vi "main_nova.vi"() -> ()   [LabVIEW 2019]
panel:
  out "error out 3":errorcluster
  in  "MoveL":bool
  out "DigitalOutput":u8[](array[numeric])
  out "DigitalInput":u8[](array[numeric])
  out "Current SpeedFactor":dbl
  out "error out 2":errorcluster
  in  "Digital Outputs Index:":i32=1 min=1 max=16 step=1
  out "Error Log":string
  in  "GetErrorID":bool
  out "x value":string
  out "y value":string
  out "z value":string
  out "rx value":string
  out "ry value":string
  out "rz value":string
  out "j6 value":string
  out "j5 value":string
  out "j4 value":string
  out "j3 value":string
  out "j2 value":string
  out "j1 value":string
  in  "rz-":bool
  in  "ry-":bool
  in  "rx-":bool
  in  "z-":bool
  in  "y-":bool
  in  "x-":bool
  in  "rz+":bool
  in  "ry+":bool
  in  "rx+":bool
  in  "z+":bool
  in  "y+":bool
  in  "x+":bool
  in  "j6":dbl
  in  "j5":dbl
  in  "j4":dbl
  in  "j3":dbl
  in  "j2":dbl
  in  "j1":dbl
  in  "Set IO confrim":bool
  in  "Status":string(combo)="1"
  in  "Feedback Port":string="30004"
  in  "Dashboard Port":string="29999"
  in  "IP Address":string="192.168.5.1"
  in  "stop get state":bool
  out "state error out 2":errorcluster
  out "Robot mode":T1(ring)
  out "speed set string":string
  in  "j6-":bool
  in  "j5-":bool
  in  "j4-":bool
  in  "j3-":bool
  in  "j2-":bool
  in  "j1-":bool
  in  "j6+":bool
  in  "j5+":bool
  in  "j4+":bool
  in  "j3+":bool
  in  "j2+":bool
  in  "j1+":bool
  in  "stop connect":bool
  in  "Start trace":bool
  in  "tracePath":string
  in  "Stop move":bool
  in  "MoveJ":bool
  in  "rz":dbl
  in  "ry":dbl
  in  "rx":dbl
  in  "z":dbl
  in  "y":dbl
  in  "x":dbl
  in  "Speed confrim":bool
  in  "Speed Ratio":dbl=50.0
  in  "Emergency Stop":bool
  in  "Power up":bool
  out "Log":string
  in  "ClearError":bool
  in  "Enable Robot":bool
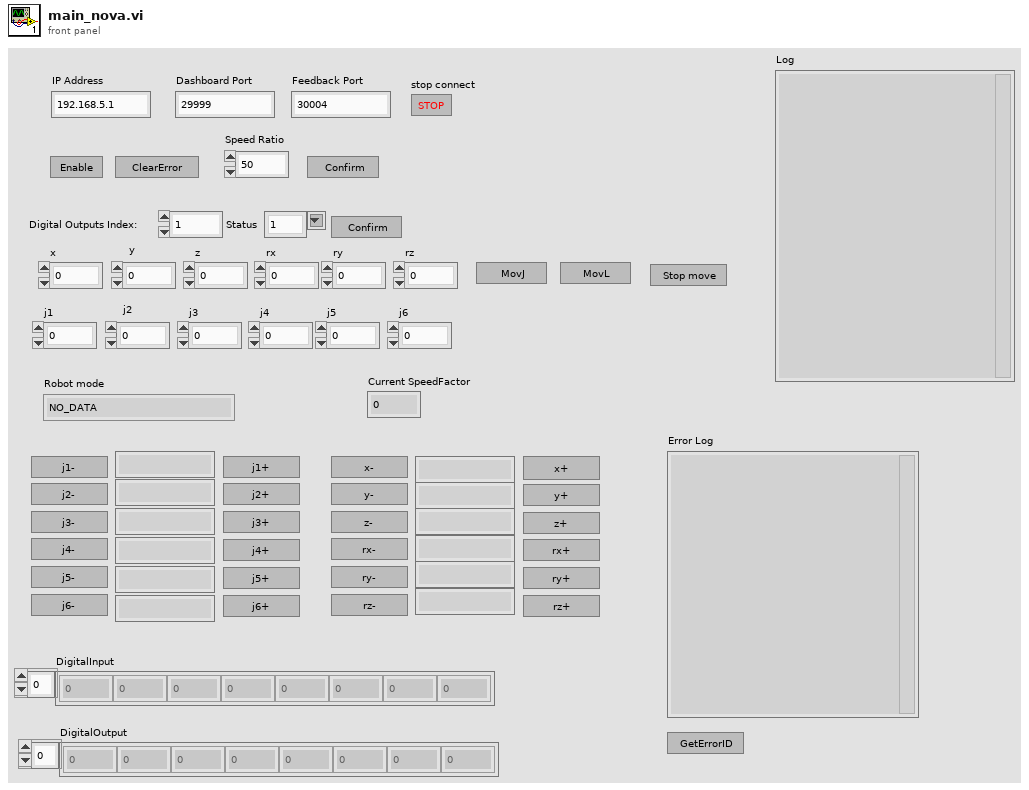
[diagram p1: front panel]
types:
  T1 = enum16{"NO_DATA", "ROBOT_MODE_INIT", "ROBOT_MODE_BRAKE_OPEN", "HOLD_BITS", "ROBOT_MODE_DISABLED", "ROBOT_MODE_ENABLE", "ROBOT_MODE_BACKDRIVE", "ROBOT_MODE_RUNNING", "ROBOT_MODE_RECORDING", "ROBOT_MODE_ERROR", "ROBOT_MODE_PAUSE", "ROBOT_MODE_JOG"}
  T2 = enum16{"Standard", "Buffered", "CRLF", "Immediate"}
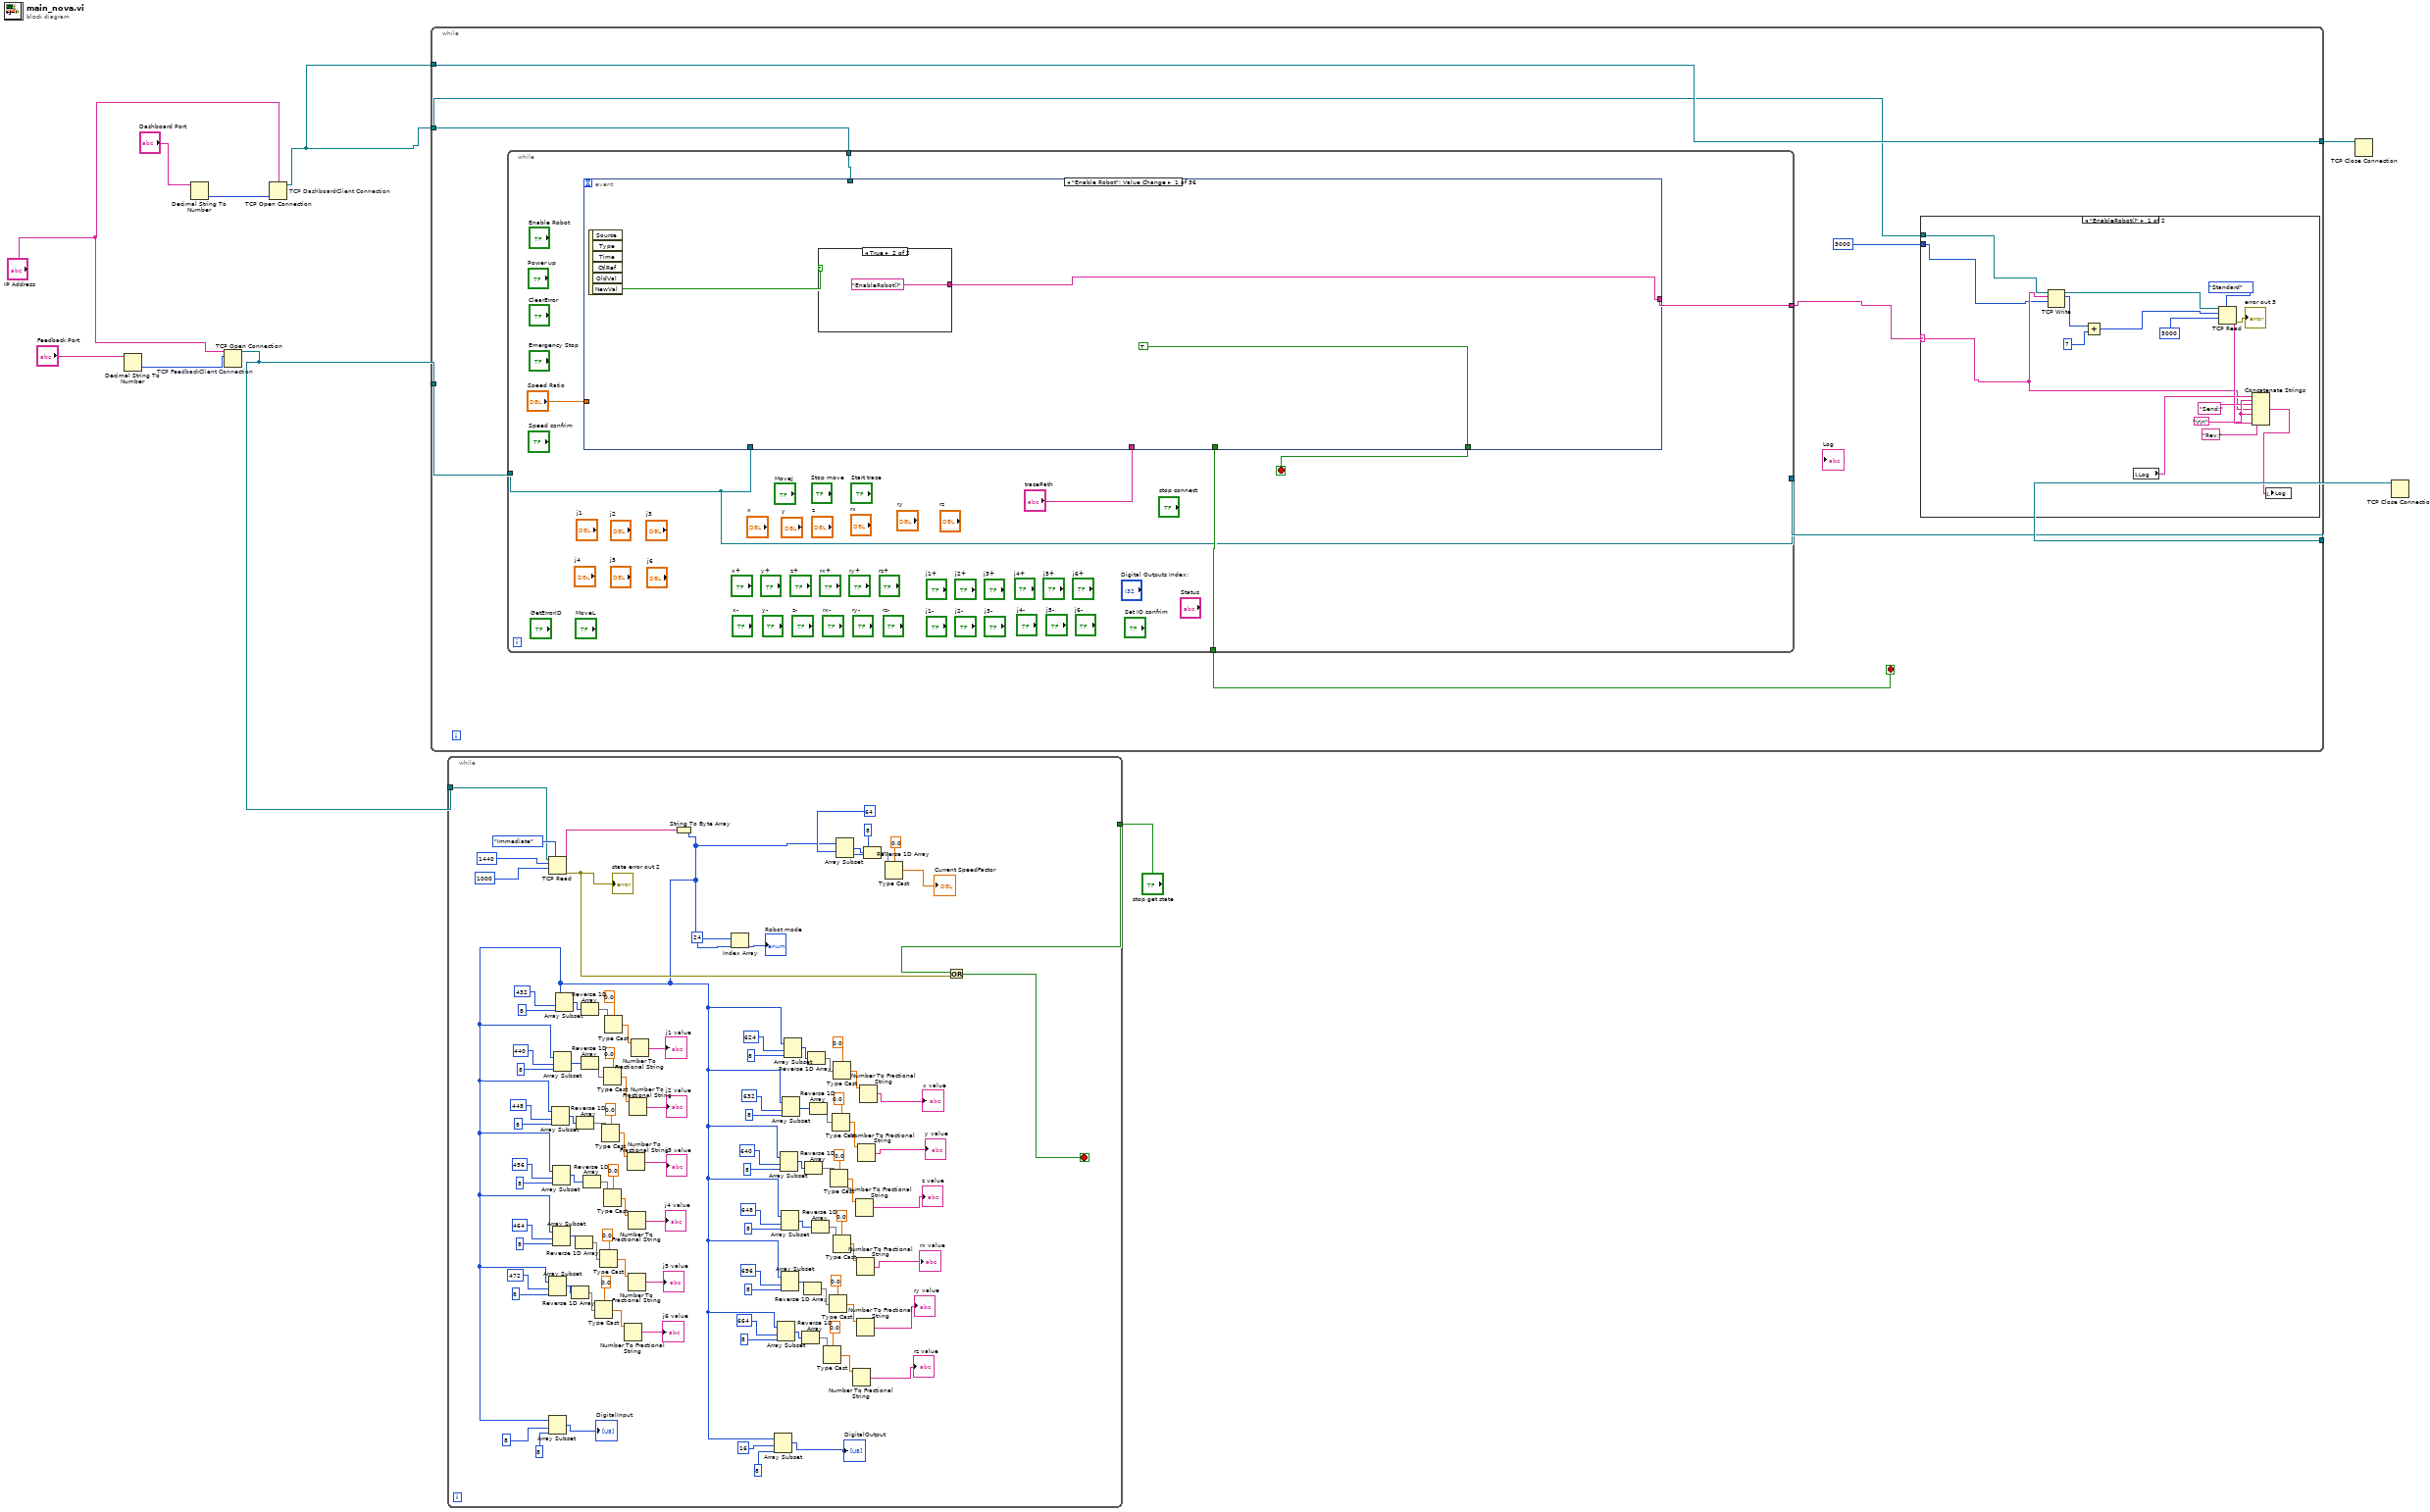
[diagram p0: block diagram]
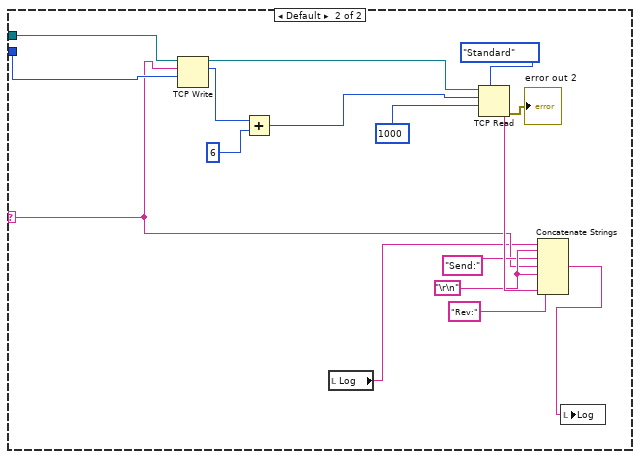
[diagram p2: hidden frame]
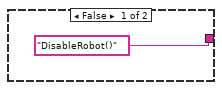
[diagram p3: hidden frame]
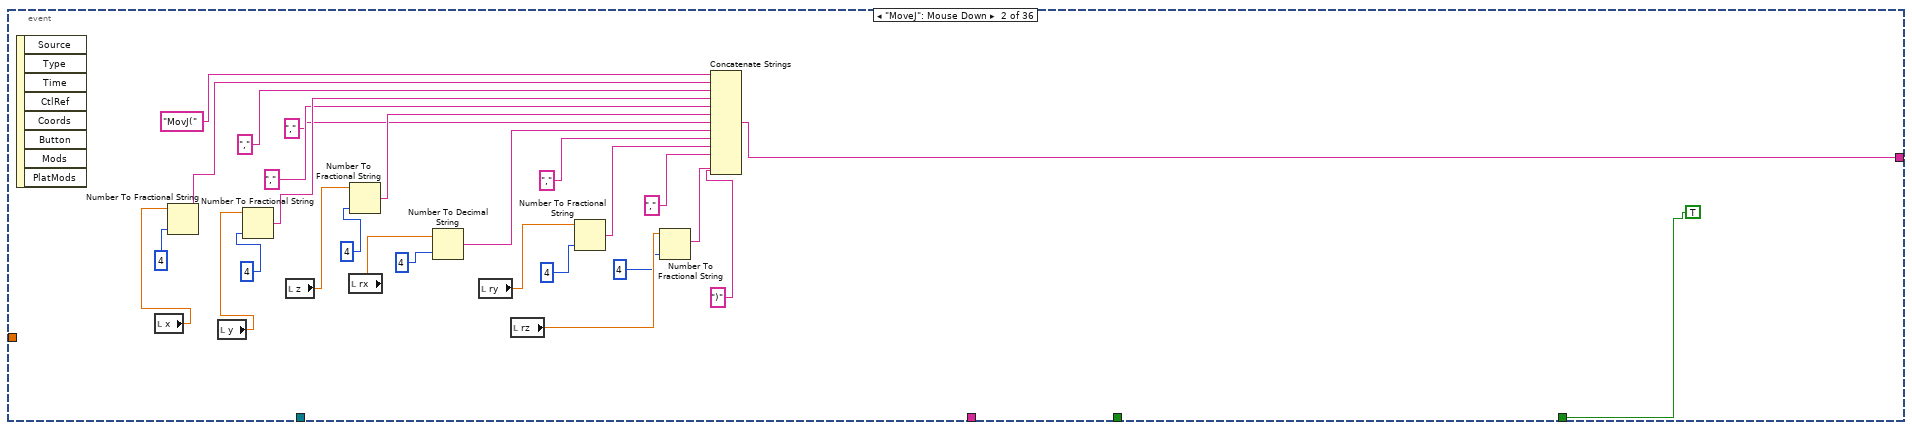
[diagram p4: hidden frame]
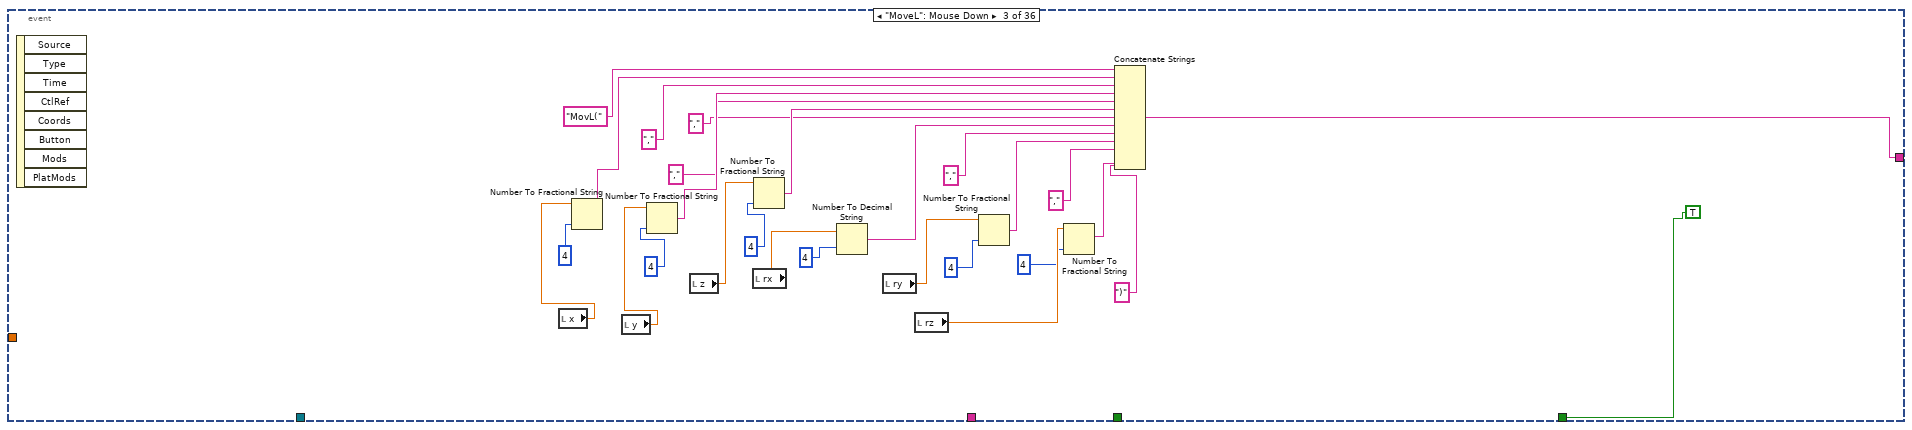
[diagram p5: hidden frame]
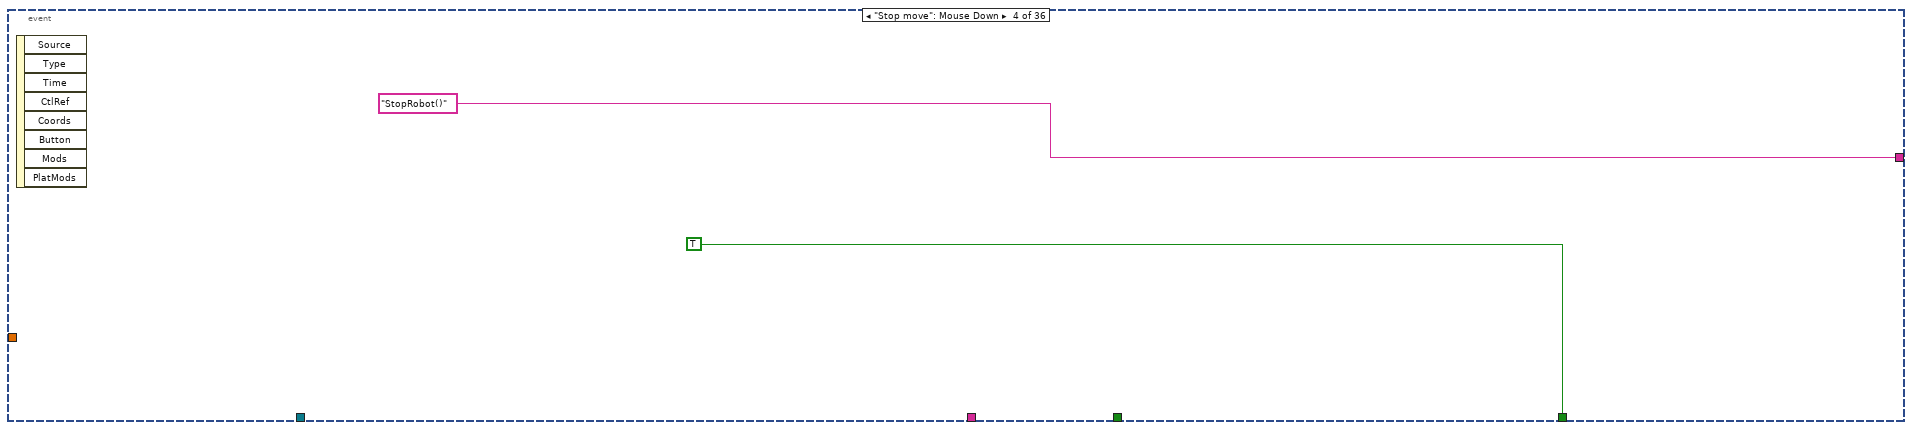
[diagram p6: hidden frame]
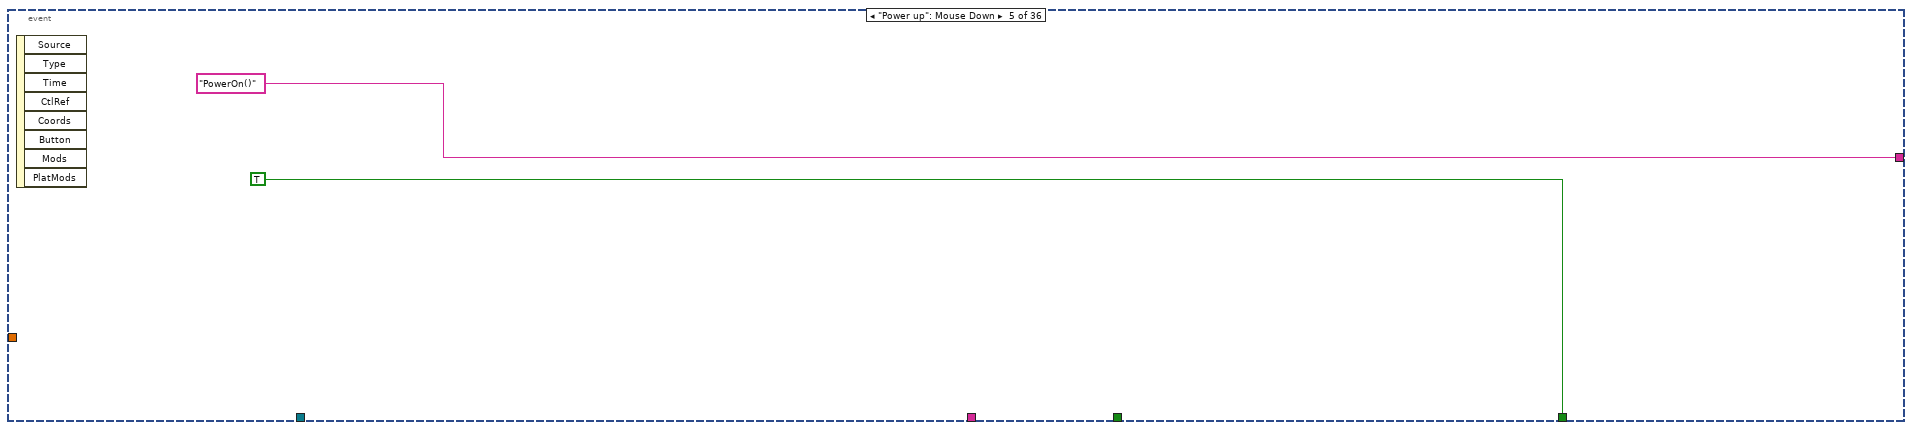
[diagram p7: hidden frame]
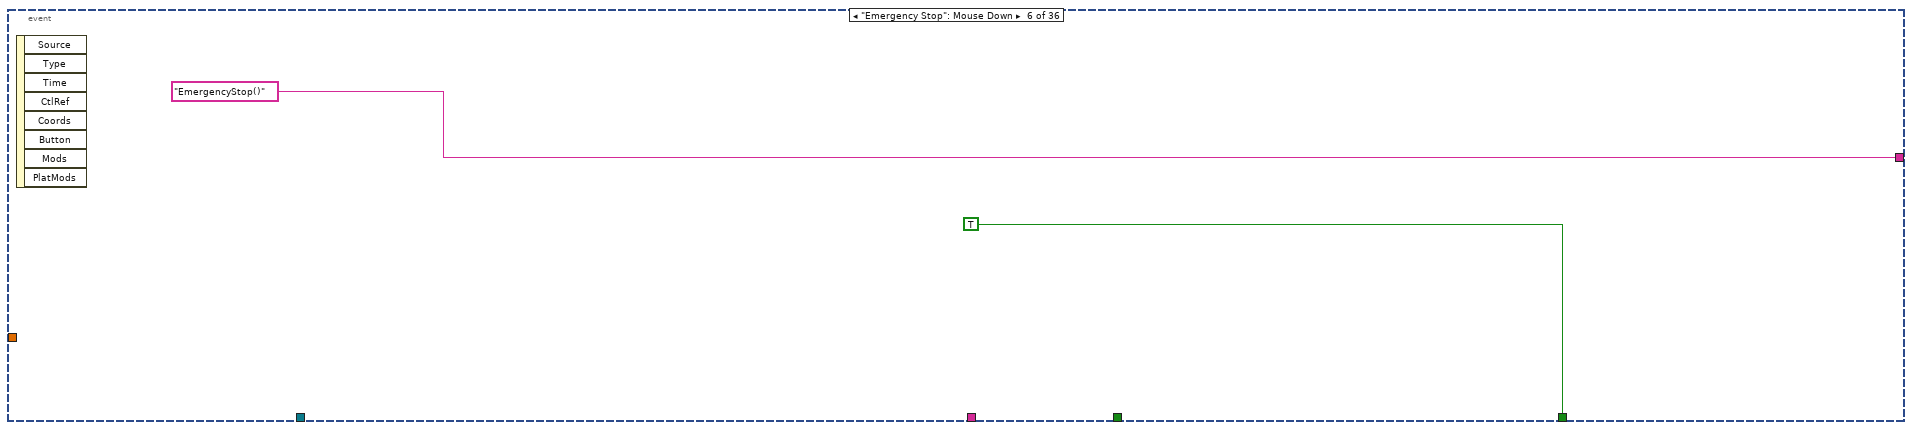
[diagram p8: hidden frame]
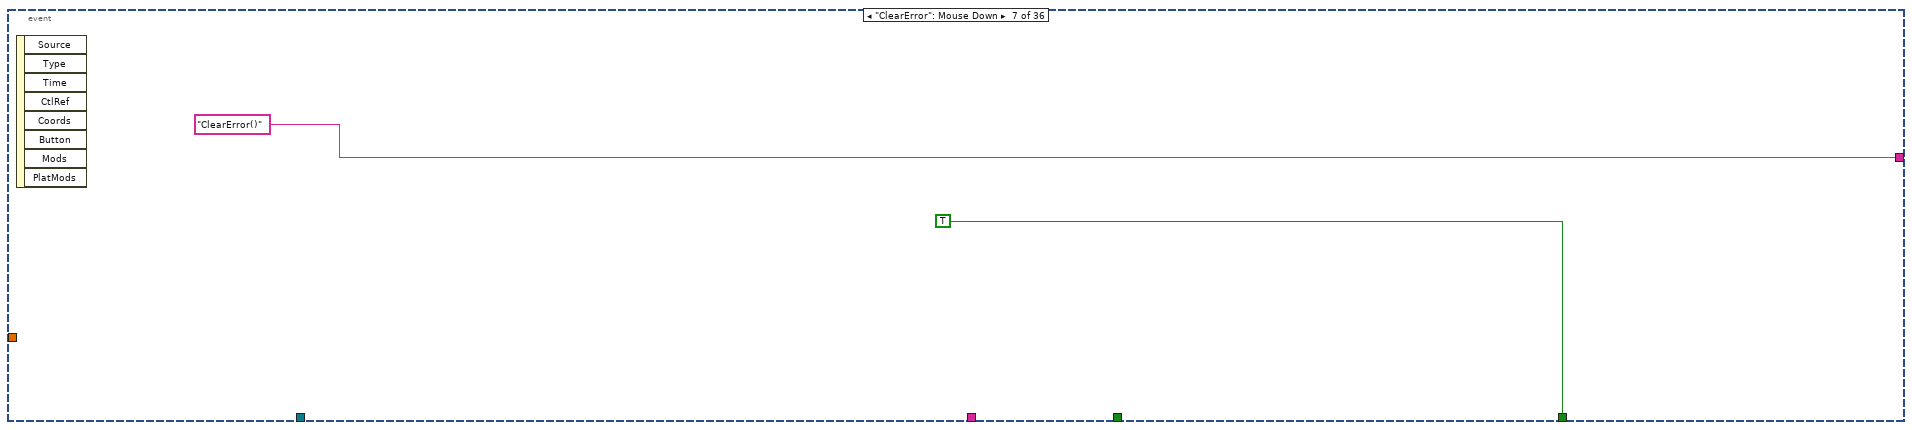
[diagram p9: hidden frame]
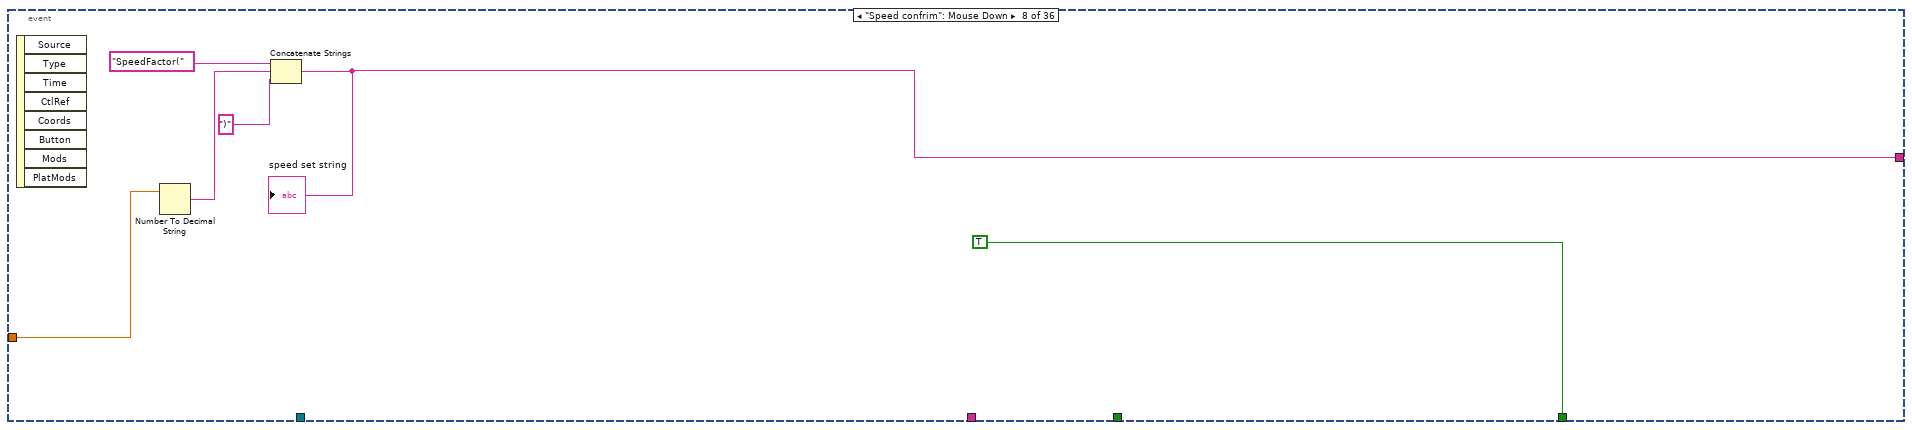
[diagram p10: hidden frame]
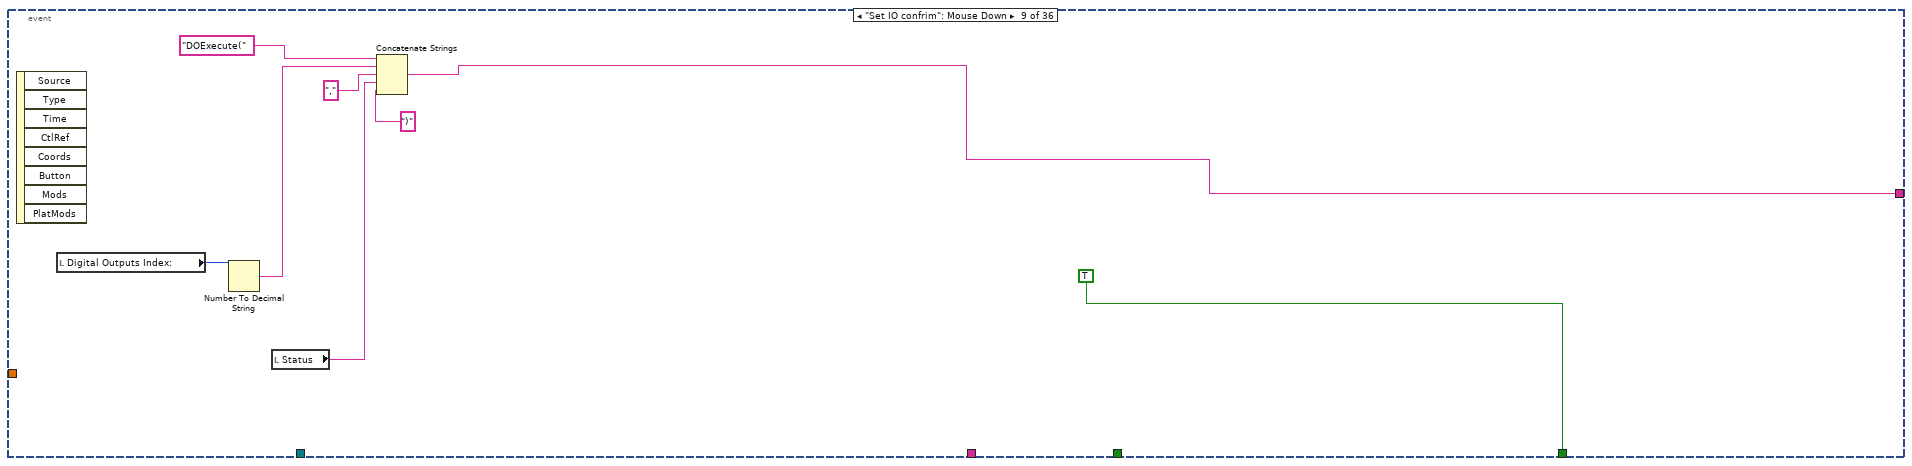
[diagram p11: hidden frame]
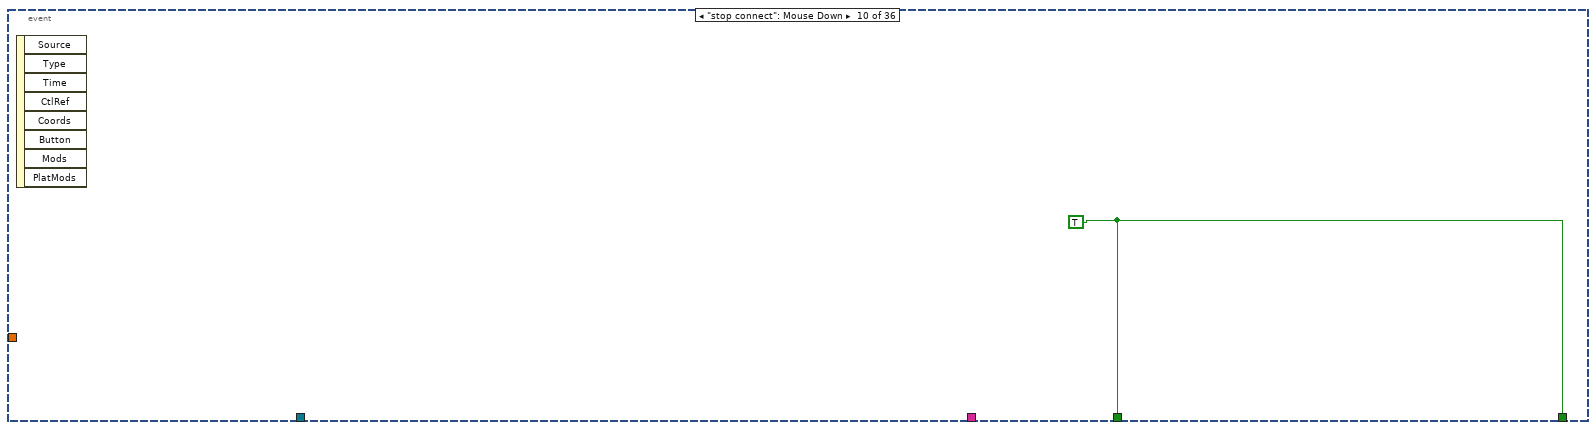
[diagram p12: hidden frame]
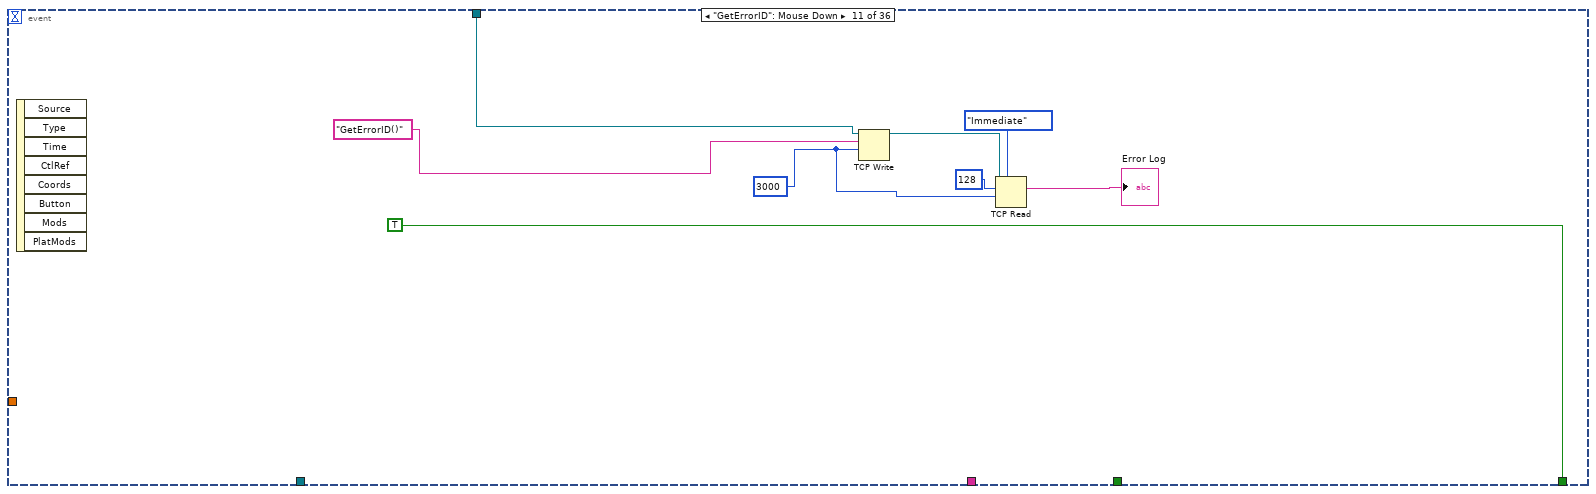
[diagram p13: hidden frame]
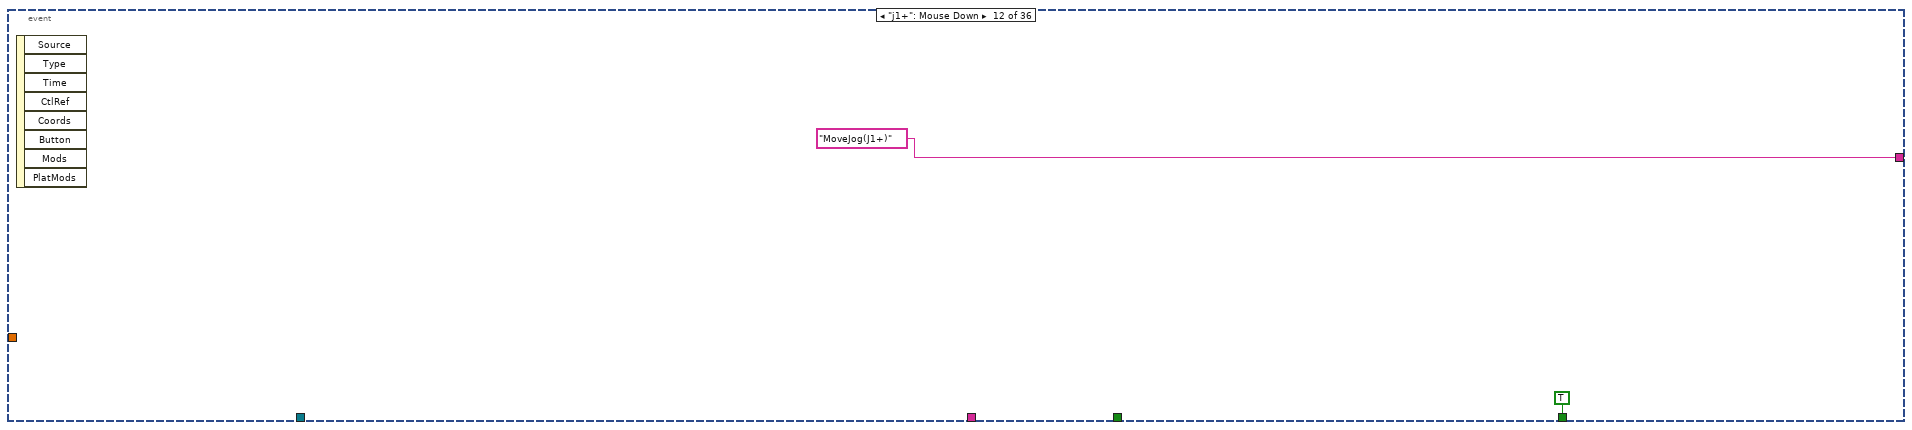
[diagram p14: hidden frame]
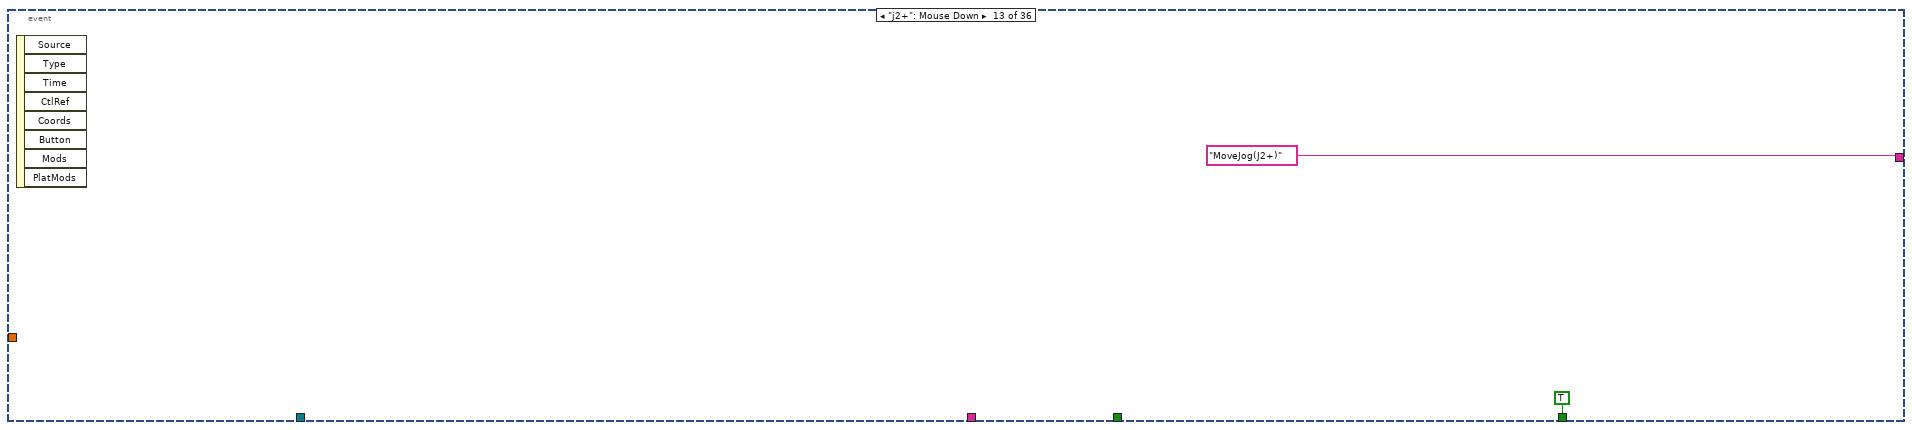
[diagram p15: hidden frame]
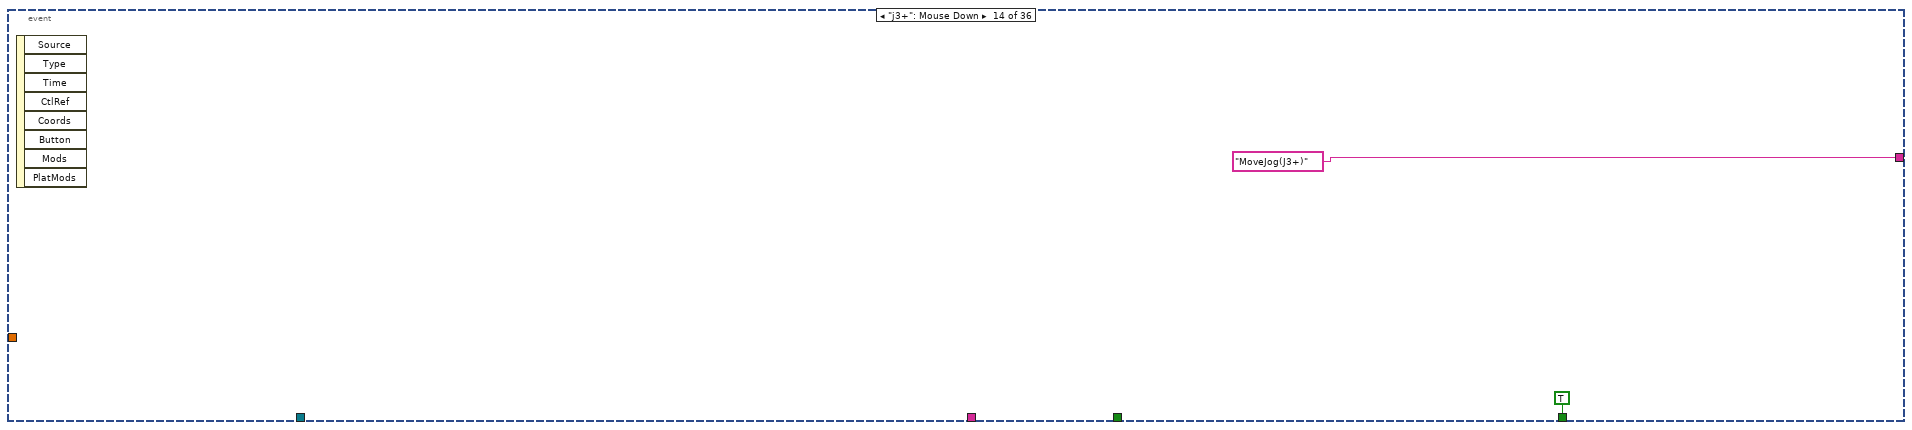
[diagram p16: hidden frame]
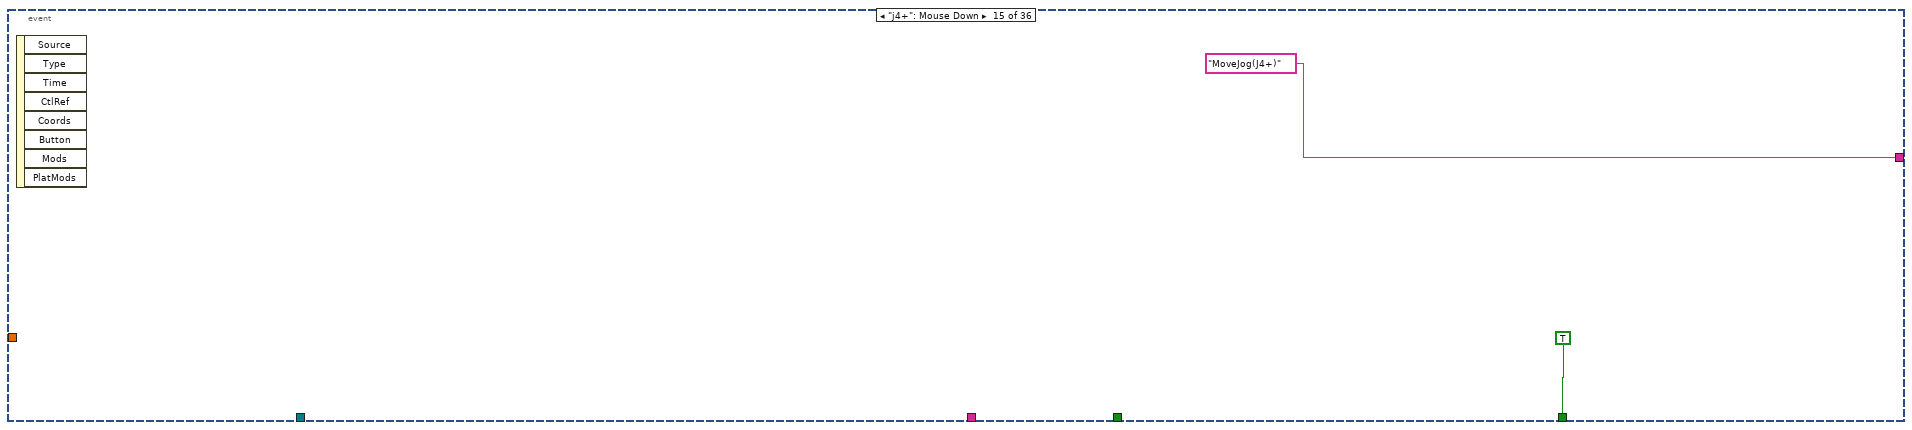
[diagram p17: hidden frame]
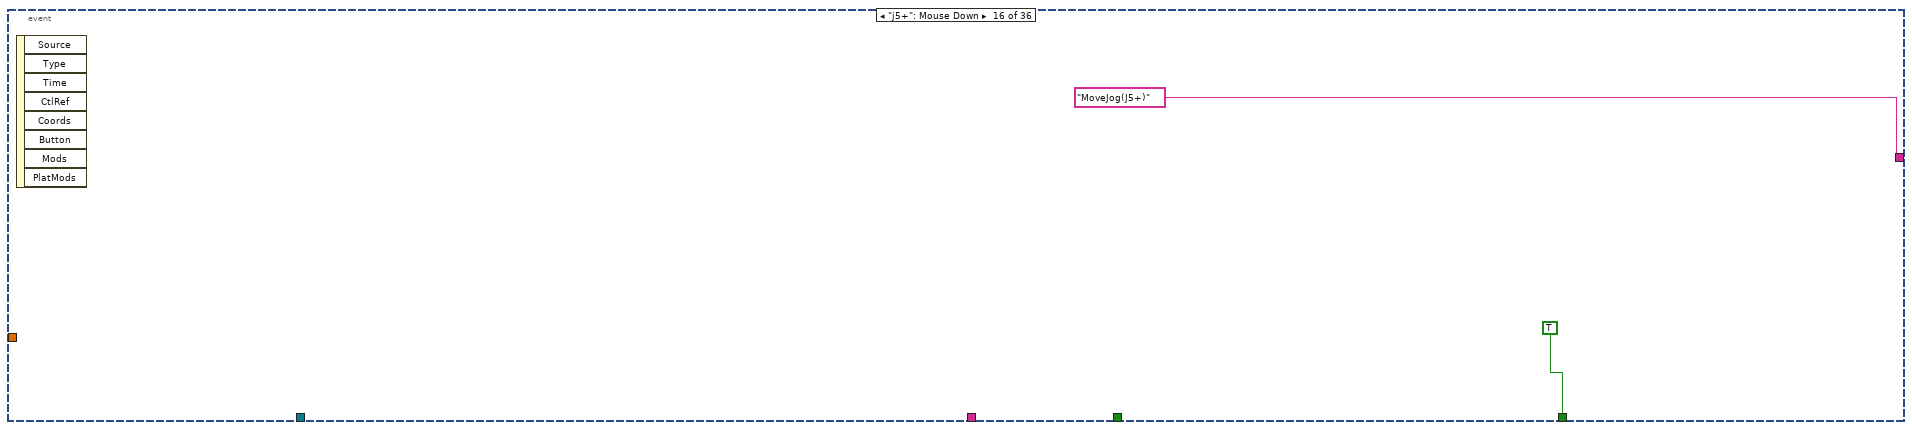
[diagram p18: hidden frame]
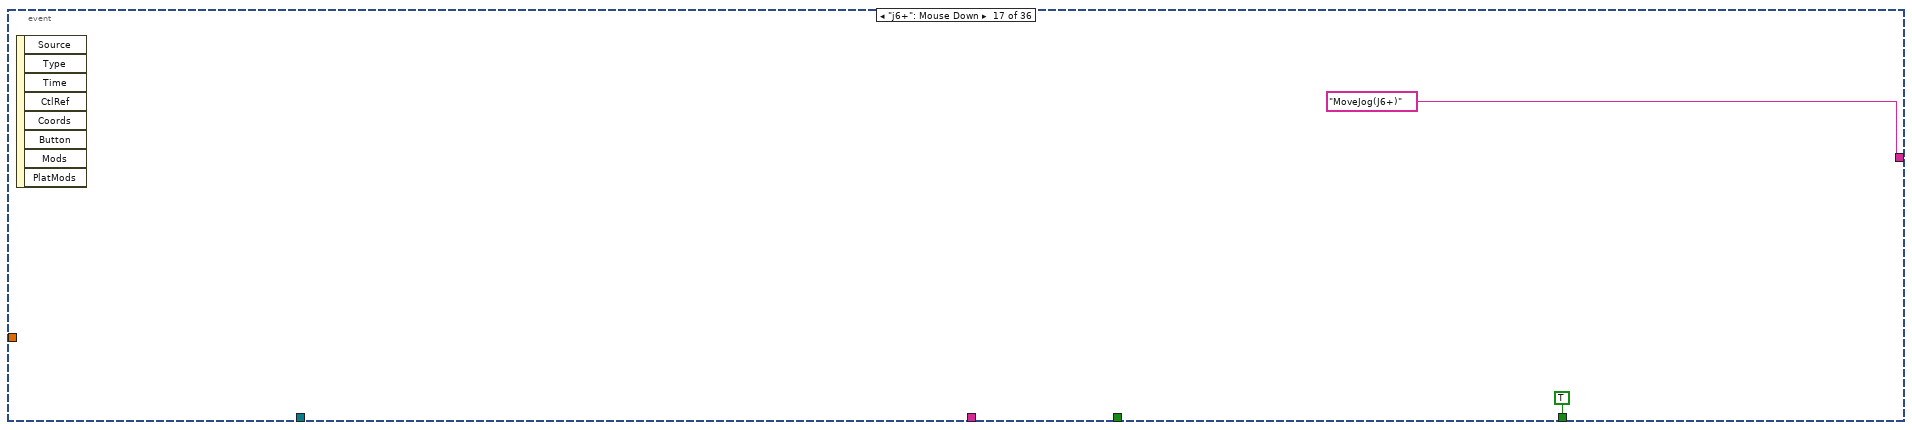
[diagram p19: hidden frame]
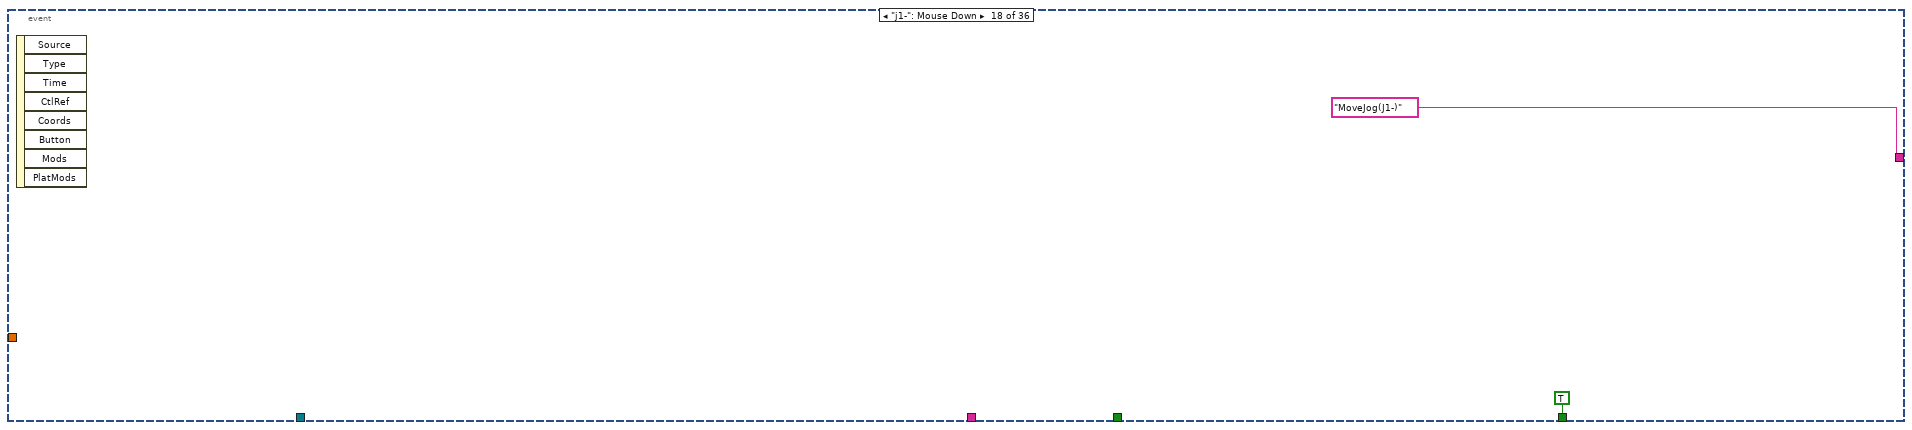
[diagram p20: hidden frame]
diagram:
  n1 = Decimal String To Number(string="Feedback Port") -> (number=w2:i32)  [unwired: 2 in, 1 out]
  n2 = Decimal String To Number(string="Dashboard Port") -> (number=w3:i32)  [unwired: 2 in, 1 out]
  n3 = TCP Open Connection "TCP FeedbackClient Connection"(address="IP Address", remote port or service name=w2) -> (connection ID=w7:refnum<k5>)  [unwired: 3 in, 1 out]
  n4 = TCP Open Connection "TCP DashboardClient Connection"(address="IP Address", remote port or service name=w3) -> (connection ID=w1:refnum<k5>)  [unwired: 3 in, 1 out]
  n5 = while {
    tunnel: [w17] -> w10
    tunnel: w1 -> [w17]
    tunnel: w7 -> [w15]
    tunnel: [w14] -> w9
    tunnel: w1 -> [w12]
    stop <- w16 stop-if-true
    n6 = while {
      tunnel: [w54] -> w16
      tunnel: w15 -> [w53]
      tunnel: [w53] -> w14
      tunnel: [w50] -> w13
      tunnel: w12 -> [w51]
      stop <- w55 stop-if-true
      n7 = event shown="[0] \"Enable Robot\": Value Change" {
        selector: _ -> [_ _ _ _ _ _ _ _ _ _ _ _ _ _ _ _ _ _ _ _ _ _ _ _ _ _ _ _ _ _ _ _ _ _ _ _]
        dyn-events: _ -> [_ _ _ _ _ _ _ _ _ _ _ _ _ _ _ _ _ _ _ _ _ _ _ _ _ _ _ _ _ _ _ _ _ _ _ _]
        timeout: _ -> [_ _ _ _ _ _ _ _ _ _ _ _ _ _ _ _ _ _ _ _ _ _ _ _ _ _ _ _ _ _ _ _ _ _ _ _]
        tunnel: [w57 w62 w89 "StopRobot()" "PowerOn()" "EmergencyStop()" "ClearError()" w125 w133 _ _ "MoveJog(J1+)" "MoveJog(J2+)" "MoveJog(J3+)" "MoveJog(J4+)" "MoveJog(J5+)" "MoveJog(J6+)" "MoveJog(J1-)" "MoveJog(J2-)" "MoveJog(J3-)" "MoveJog(J4-)" "MoveJog(J5-)" "MoveJog(J6-)" "MoveJog(X+)" "MoveJog(Y+)" "MoveJog(Z+)" "MoveJog(Rx+)" "MoveJog(Ry+)" "MoveJog(Rz+)" "MoveJog(X-)" "MoveJog(Y-)" "MoveJog(Z-)" "MoveJog(Rx-)" "MoveJog(Ry-)" "MoveJog(Rz-)" "MoveJog()"] -> w50
        tunnel: "tracePath" -> [_ _ _ _ _ _ _ _ _ _ _ _ _ _ _ _ _ _ _ _ _ _ _ _ _ _ _ _ _ _ _ _ _ _ _ _]
        tunnel: [TRUE TRUE TRUE TRUE TRUE TRUE TRUE TRUE TRUE w138 TRUE TRUE TRUE TRUE TRUE TRUE TRUE TRUE TRUE TRUE TRUE TRUE TRUE TRUE TRUE TRUE TRUE TRUE TRUE TRUE TRUE TRUE TRUE TRUE TRUE TRUE] -> w55
        tunnel: [_ _ _ _ _ _ _ _ _ w138 _ _ _ _ _ _ _ _ _ _ _ _ _ _ _ _ _ _ _ _ _ _ _ _ _ _] -> w54
        tunnel: w53 -> [_ _ _ _ _ _ _ _ _ _ _ _ _ _ _ _ _ _ _ _ _ _ _ _ _ _ _ _ _ _ _ _ _ _ _ _]
        tunnel: "Speed Ratio" -> [_ _ _ _ _ _ _ w124 _ _ _ _ _ _ _ _ _ _ _ _ _ _ _ _ _ _ _ _ _ _ _ _ _ _ _ _]
        tunnel: w51 -> [_ _ _ _ _ _ _ _ _ _ w139 _ _ _ _ _ _ _ _ _ _ _ _ _ _ _ _ _ _ _ _ _ _ _ _ _]
        event "Enable Robot": Value Change {
          n8 = event-data() -> ("NewVal"=w59:bool)  [unwired: 1 in, 5 out]
          n9 = case shown="True" w59 {
            tunnel: ["DisableRobot()" "EnableRobot()"] -> w57
            frame False {
            }
            frame True {
            }
          }
        }
        event "MoveJ": Mouse Down {
          n10 = event-data() -> ()  [unwired: 1 in, 8 out]
          n11 = local read "x"() -> (w63:dbl)
          n12 = Number To Fractional String(number=w63, precision (6)=i16 4) -> (F-format string=w77:string)  [unwired: 2 in]
          n13 = local read "y"() -> (w87:dbl)
          n14 = Number To Fractional String(number=w87, precision (6)=i16 4) -> (F-format string=w78:string)  [unwired: 2 in]
          n15 = local read "z"() -> (w86:dbl)
          n16 = local read "rx"() -> (w85:dbl)
          n17 = Number To Fractional String(number=w86, precision (6)=i16 4) -> (F-format string=w82:string)  [unwired: 2 in]
          n18 = Number To Decimal String(number=w85, width (-)=i16 4 ("precision (6)")) -> (decimal integer string=w79:string)
          n19 = local read "ry"() -> (w84:dbl)
          n20 = local read "rz"() -> (w83:dbl)
          n21 = Number To Fractional String(number=w84, precision (6)=i16 4) -> (F-format string=w80:string)  [unwired: 2 in]
          n22 = Number To Fractional String(number=w83, precision (6)=i16 4) -> (F-format string=w81:string)  [unwired: 2 in]
          n23 = Concatenate Strings("MovJ(" ("string"), w77, "," ("string"), w78, "," ("string"), w82, "," ("string"), w79, "," ("string"), w80, "," ("string"), w81, ")" ("string")) -> (w62:string)
        }
        event "MoveL": Mouse Down {
          n24 = event-data() -> ()  [unwired: 1 in, 8 out]
          n25 = local read "x"() -> (w114:dbl)
          n26 = Number To Fractional String(number=w114, precision (6)=i16 4) -> (F-format string=w103:string)  [unwired: 2 in]
          n27 = local read "y"() -> (w113:dbl)
          n28 = Number To Fractional String(number=w113, precision (6)=i16 4) -> (F-format string=w104:string)  [unwired: 2 in]
          n29 = local read "z"() -> (w112:dbl)
          n30 = local read "rx"() -> (w111:dbl)
          n31 = Number To Fractional String(number=w112, precision (6)=i16 4) -> (F-format string=w108:string)  [unwired: 2 in]
          n32 = Number To Decimal String(number=w111, width (-)=i16 4 ("precision (6)")) -> (decimal integer string=w105:string)
          n33 = local read "ry"() -> (w110:dbl)
          n34 = local read "rz"() -> (w109:dbl)
          n35 = Number To Fractional String(number=w110, precision (6)=i16 4) -> (F-format string=w106:string)  [unwired: 2 in]
          n36 = Number To Fractional String(number=w109, precision (6)=i16 4) -> (F-format string=w107:string)  [unwired: 2 in]
          n37 = Concatenate Strings("MovL(" ("string"), w103, "," ("string"), w104, "," ("string"), w108, "," ("string"), w105, "," ("string"), w106, "," ("string"), w107, ")" ("string")) -> (w89:string)
        }
        event "Stop move": Mouse Down {
          n38 = event-data() -> ()  [unwired: 1 in, 8 out]
        }
        event "Power up": Mouse Down {
          n39 = event-data() -> ()  [unwired: 1 in, 8 out]
        }
        event "Emergency Stop": Mouse Down {
          n40 = event-data() -> ()  [unwired: 1 in, 8 out]
        }
        event "ClearError": Mouse Down {
          n41 = event-data() -> ()  [unwired: 1 in, 8 out]
        }
        event "Speed confrim": Mouse Down {
          n42 = event-data() -> ()  [unwired: 1 in, 8 out]
          n43 = Number To Decimal String(number=w124) -> (decimal integer string=w129:string)  [unwired: 1 in]
          n44 = Concatenate Strings("SpeedFactor(", w129, ")") -> (w125:string)
          "speed set string" <- w125
        }
        event "Set IO confrim": Mouse Down {
          n45 = event-data() -> ()  [unwired: 1 in, 8 out]
          n46 = local read "Digital Outputs Index:"() -> (w131:i32)
          n47 = Number To Decimal String(number=w131) -> (decimal integer string=w137:string)  [unwired: 1 in]
          n48 = local read "Status"() -> (w130:string)
          n49 = Concatenate Strings("DOExecute(", w137, "," ("string"), w130, ")") -> (w133:string)
        }
        event "stop connect": Mouse Down {
          w138 = TRUE
          n50 = event-data() -> ()  [unwired: 1 in, 8 out]
        }
        event "GetErrorID": Mouse Down {
          w143 = 3000 ("timeout ms (25000)")
          n51 = event-data() -> ()  [unwired: 1 in, 8 out]
          n52 = TCP Write(connection ID=w139, data in="GetErrorID()", 9:w143) -> (connection ID out=w144:refnum<k5>)  [unwired: 1 in, 2 out]
          n53 = TCP Read(connection ID=w144, bytes to read=128, 7:T2."Immediate" ("mode (standard)"), 9:w143) -> (data out=→"Error Log":string)  [unwired: 1 in, 2 out]
        }
        event "j1+": Mouse Down {
          n54 = event-data() -> ()  [unwired: 1 in, 8 out]
        }
        event "j2+": Mouse Down {
          n55 = event-data() -> ()  [unwired: 1 in, 8 out]
        }
        event "j3+": Mouse Down {
          n56 = event-data() -> ()  [unwired: 1 in, 8 out]
        }
        event "j4+": Mouse Down {
          n57 = event-data() -> ()  [unwired: 1 in, 8 out]
        }
        event "j5+": Mouse Down {
          n58 = event-data() -> ()  [unwired: 1 in, 8 out]
        }
        event "j6+": Mouse Down {
          n59 = event-data() -> ()  [unwired: 1 in, 8 out]
        }
        event "j1-": Mouse Down {
          n60 = event-data() -> ()  [unwired: 1 in, 8 out]
        }
        event "j2-": Mouse Down {
          n61 = event-data() -> ()  [unwired: 1 in, 8 out]
        }
        event "j3-": Mouse Down {
          n62 = event-data() -> ()  [unwired: 1 in, 8 out]
        }
        event "j4-": Mouse Down {
          n63 = event-data() -> ()  [unwired: 1 in, 8 out]
        }
        event "j5-": Mouse Down {
          n64 = event-data() -> ()  [unwired: 1 in, 8 out]
        }
        event "j6-": Mouse Down {
          n65 = event-data() -> ()  [unwired: 1 in, 8 out]
        }
        event "x+": Mouse Down {
          n66 = event-data() -> ()  [unwired: 1 in, 8 out]
        }
        event "y+": Mouse Down {
          n67 = event-data() -> ()  [unwired: 1 in, 8 out]
        }
        event "z+": Mouse Down {
          n68 = event-data() -> ()  [unwired: 1 in, 8 out]
        }
        event "rx+": Mouse Down {
          n69 = event-data() -> ()  [unwired: 1 in, 8 out]
        }
        event "ry+": Mouse Down {
          n70 = event-data() -> ()  [unwired: 1 in, 8 out]
        }
        event "rz+": Mouse Down {
          n71 = event-data() -> ()  [unwired: 1 in, 8 out]
        }
        event "x-": Mouse Down {
          n72 = event-data() -> ()  [unwired: 1 in, 8 out]
        }
        event "y-": Mouse Down {
          n73 = event-data() -> ()  [unwired: 1 in, 8 out]
        }
        event "z-": Mouse Down {
          n74 = event-data() -> ()  [unwired: 1 in, 8 out]
        }
        event "rx-": Mouse Down {
          n75 = event-data() -> ()  [unwired: 1 in, 8 out]
        }
        event "ry-": Mouse Down {
          n76 = event-data() -> ()  [unwired: 1 in, 8 out]
        }
        event "rz-": Mouse Down {
          n77 = event-data() -> ()  [unwired: 1 in, 8 out]
        }
        event "j6-", "j2+", "j3+", "j4+", "j5+", "j6+", "j1-", "j2-", "j3-", "j4-", "j5-", "x+", "y+", "z+", "rx+", "ry+", "rz+", "x-", "y-", "z-", "rx-", "ry-", "rz-", "j1+": Mouse Up {
          n78 = event-data() -> ()  [unwired: 1 in, 8 out]
        }
      }
    }
    n79 = case shown="\"EnableRobot()\"" w13 {
      tunnel: 3000 ("timeout ms (25000)") -> [w19 w41]
      tunnel: w12 -> [w18 w40]
      selector: w13 -> [w20 w39]
      frame "EnableRobot()" {
        w30 = "\r\n"
        n80 = TCP Write(connection ID=w18, data in=w20, 9:w19) -> (connection ID out=w31:refnum<k5>, bytes written=w23:i32)  [unwired: 1 in, 1 out]
        n81 = Add(x=w23, y=7) -> (x+y=w22:i32)
        n82 = local read "Log"() -> (w24:string)
        n83 = TCP Read(connection ID=w31, bytes to read=w22, 7:T2."Standard" ("mode (standard)"), 9:3000 ("timeout ms (25000)")) -> (data out=w32:string, error out=→"error out 3":errorcluster)  [unwired: 1 in, 1 out]
        n84 = Concatenate Strings(w24, w30, "Send:" ("string"), w20, w30, "Rev:" ("string"), w32) -> (w25:string)
        n85 = local write "Log"(w25) -> ()
      }
      frame Default {
        w46 = "\r\n"
        n86 = TCP Write(connection ID=w40, data in=w39, 9:w41) -> (connection ID out=w47:refnum<k5>, bytes written=w36:i32)  [unwired: 1 in, 1 out]
        n87 = Add(x=w36, y=6) -> (x+y=w35:i32)
        n88 = local read "Log"() -> (w37:string)
        n89 = TCP Read(connection ID=w47, bytes to read=w35, 7:T2."Standard" ("mode (standard)"), 9:1000 ("timeout ms (25000)")) -> (data out=w48:string, error out=→"error out 2":errorcluster)  [unwired: 1 in, 1 out]
        n90 = Concatenate Strings(w37, w46, "Send:" ("string"), w39, w46, "Rev:" ("string"), w48) -> (w38:string)
        n91 = local write "Log"(w38) -> ()
      }
    }
  }
  n92 = while {
    tunnel: w7 -> [w300]
    tunnel: "stop get state" -> [w297]
    stop <- w296 stop-if-true
    n93 = TCP Read(connection ID=w300, bytes to read=1440, 7:T2."Immediate" ("mode (standard)"), 9:1000 ("timeout ms (25000)")) -> (data out=w298:string, error out=w295:errorcluster)  [unwired: 1 in, 1 out]
    "state error out 2" <- w295
    n94 = String To Byte Array(string=w298) -> (unsigned byte array=w199:u8[])
    n95 = Array Subset(array=w199, index=472, length=8) -> (w214:u8[])
    n96 = Array Subset(array=w199, index=8, length=8) -> (→"DigitalInput":u8[])
    n97 = Array Subset(array=w199, index=448, length=8) -> (w260:u8[])
    n98 = Array Subset(array=w199, index=456, length=8) -> (w258:u8[])
    n99 = Array Subset(array=w199, index=464, length=8) -> (w256:u8[])
    n100 = Array Subset(array=w199, index=440, length=8) -> (w261:u8[])
    n101 = Array Subset(array=w199, index=432, length=8) -> (w264:u8[])
    n102 = Reverse 1D Array(array=w214) -> (reversed array=w213:u8[])
    n103 = Reverse 1D Array(array=w256) -> (reversed array=w255:u8[])
    n104 = Reverse 1D Array(array=w260) -> (reversed array=w259:u8[])
    n105 = Reverse 1D Array(array=w264) -> (reversed array=w263:u8[])
    n106 = Reverse 1D Array(array=w261) -> (reversed array=w262:u8[])
    n107 = Reverse 1D Array(array=w258) -> (reversed array=w257:u8[])
    n108 = Type Cast(type=0.0, x=w213) -> (*(type *) &x=w269:dbl)
    n109 = Type Cast(type=0.0, x=w255) -> (*(type *) &x=w273:dbl)
    n110 = Type Cast(type=0.0, x=w259) -> (*(type *) &x=w281:dbl)
    n111 = Type Cast(type=0.0, x=w262) -> (*(type *) &x=w286:dbl)
    n112 = Type Cast(type=0.0, x=w257) -> (*(type *) &x=w277:dbl)
    n113 = Type Cast(type=0.0, x=w263) -> (*(type *) &x=w291:dbl)
    n114 = Number To Fractional String(number=w269) -> (F-format string=→"j6 value":string)  [unwired: 3 in]
    n115 = Number To Fractional String(number=w281) -> (F-format string=→"j3 value":string)  [unwired: 3 in]
    n116 = Number To Fractional String(number=w277) -> (F-format string=→"j4 value":string)  [unwired: 3 in]
    n117 = Number To Fractional String(number=w273) -> (F-format string=→"j5 value":string)  [unwired: 3 in]
    n118 = Number To Fractional String(number=w286) -> (F-format string=→"j2 value":string)  [unwired: 3 in]
    n119 = Number To Fractional String(number=w291) -> (F-format string=→"j1 value":string)  [unwired: 3 in]
    n120 = Index Array(array=w199, index=24) -> (element=→"Robot mode":u8)
    n121 = Array Subset(array=w199, index=16, length=8) -> (→"DigitalOutput":u8[])
    n122 = Array Subset(array=w199, index=664, length=8) -> (w212:u8[])
    n123 = Array Subset(array=w199, index=640, length=8) -> (w228:u8[])
    n124 = Array Subset(array=w199, index=648, length=8) -> (w226:u8[])
    n125 = Array Subset(array=w199, index=656, length=8) -> (w224:u8[])
    n126 = Array Subset(array=w199, index=632, length=8) -> (w229:u8[])
    n127 = Array Subset(array=w199, index=624, length=8) -> (w216:u8[])
    n128 = Reverse 1D Array(array=w212) -> (reversed array=w211:u8[])
    n129 = Reverse 1D Array(array=w224) -> (reversed array=w223:u8[])
    n130 = Reverse 1D Array(array=w228) -> (reversed array=w227:u8[])
    n131 = Reverse 1D Array(array=w216) -> (reversed array=w215:u8[])
    n132 = Reverse 1D Array(array=w229) -> (reversed array=w230:u8[])
    n133 = Reverse 1D Array(array=w226) -> (reversed array=w225:u8[])
    n134 = Type Cast(type=0.0, x=w211) -> (*(type *) &x=w231:dbl)
    n135 = Type Cast(type=0.0, x=w223) -> (*(type *) &x=w235:dbl)
    n136 = Type Cast(type=0.0, x=w227) -> (*(type *) &x=w243:dbl)
    n137 = Type Cast(type=0.0, x=w230) -> (*(type *) &x=w247:dbl)
    n138 = Type Cast(type=0.0, x=w225) -> (*(type *) &x=w239:dbl)
    n139 = Type Cast(type=0.0, x=w215) -> (*(type *) &x=w251:dbl)
    n140 = Array Subset(array=w199, index=64, length=8) -> (w206:u8[])
    n141 = Number To Fractional String(number=w231) -> (F-format string=→"rz value":string)  [unwired: 3 in]
    n142 = Number To Fractional String(number=w243) -> (F-format string=→"z value":string)  [unwired: 3 in]
    n143 = Number To Fractional String(number=w239) -> (F-format string=→"rx value":string)  [unwired: 3 in]
    n144 = Number To Fractional String(number=w235) -> (F-format string=→"ry value":string)  [unwired: 3 in]
    n145 = Number To Fractional String(number=w247) -> (F-format string=→"y value":string)  [unwired: 3 in]
    n146 = Number To Fractional String(number=w251) -> (F-format string=→"x value":string)  [unwired: 3 in]
    n147 = Reverse 1D Array(array=w206) -> (reversed array=w205:u8[])
    n148 = Type Cast(type=0.0, x=w205) -> (*(type *) &x=→"Current SpeedFactor":dbl)
    n149 = Or(x=w297, y=w295) -> (x .or. y?=w296:bool)
  }
  n150 = TCP Close Connection(connection ID=w10) -> ()  [unwired: 2 in, 2 out]
  n151 = TCP Close Connection(connection ID=w9) -> ()  [unwired: 2 in, 2 out]
